vi "retraceSearchPath.vi"(8 "error in (no error)":errorcluster, 10 "GoalNode":refnum<data-value>, 11 "Graph in":refnum<class "Graph.lvclass">) -> (0 "error out":errorcluster, 2 "SearchPath":refnum<data-value>[](array[refnum]), 3 "Graph out":refnum<class "Graph.lvclass">)   [LabVIEW 2010, in "Graph.lvclass"]
doc: "At the end of a search, we retrace the path it took to reach the goal node."
uses:
  Graph.lvclass
  GraphNode/GraphNode.lvclass
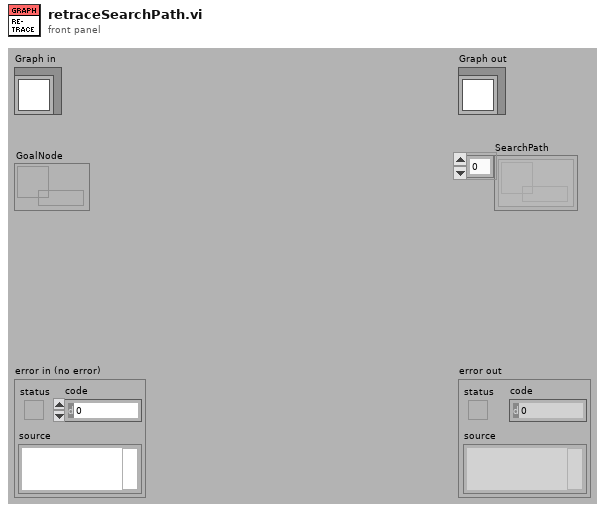
[diagram p1: front panel]
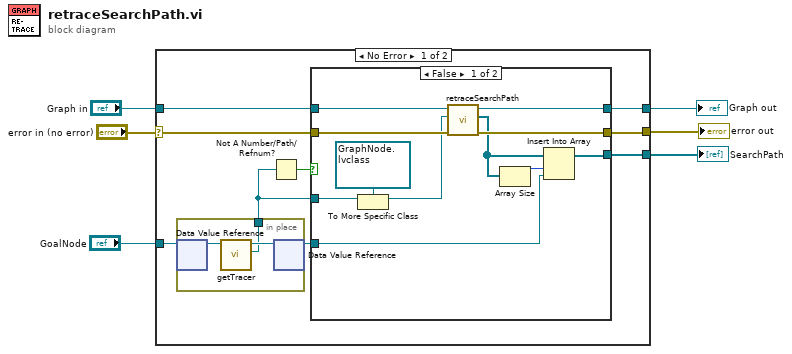
[diagram p0: block diagram]
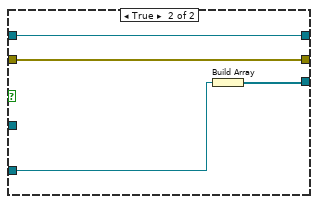
[diagram p2: hidden frame]
diagram:
  n1 = case shown="No Error" "error in (no error)" {
    selector: "error in (no error)" -> [w13 w35]
    tunnel: [w11 w35] -> w5
    tunnel: [w14 w34] -> w3
    tunnel: "Graph in" -> [w15 w34]
    tunnel: "GoalNode" -> [w12 _]
    tunnel: [w10 _] -> w1
    frame No Error {
      n2 = in-place {
        in-place-border: [w31] -> w7
        n3 = in-place-dvr #1(w12) -> (w33:refnum<class "GraphNode.lvclass">)  [unwired: 1 out]
        n4 = call "getTracer.vi"("GraphNode in"=w33) -> ("tracer"=w31:refnum<data-value>, "GraphNode out"=w32:refnum<class "GraphNode.lvclass">)  [unwired: 8 in, 1 out]
        n5 = in-place-dvr #1(w32) -> (w9:refnum<data-value>)  [unwired: 1 out]
      }
      n6 = Not A Number/Path/Refnum?(number/path/refnum=w7) -> (NaN/Path/Refnum?=w8:bool)
      n7 = case shown="False" w8 {
        tunnel: w15 -> [w26 w27]
        tunnel: [w25 w27] -> w14
        tunnel: w13 -> [w24 w28]
        tunnel: [w23 w28] -> w11
        tunnel: [w22 w29] -> w10
        tunnel: w9 -> [w19 w30]
        tunnel: w7 -> [w18 _]
        frame False {
          n8 = To More Specific Class(target class=refnum<data-value> refnum ("GoalNode"), reference=w18) -> (specific class reference=w20:refnum<data-value>)  [unwired: 1 in, 1 out]
          n9 = call "retraceSearchPath.vi"("error in (no error)"=w24, "GoalNode"=w20, "Graph in"=w26) -> ("error out"=w23:errorcluster, "SearchPath"=w17:refnum<data-value>[], "Graph out"=w25:refnum<class "Graph.lvclass">)  [unwired: 6 in]
          n10 = Array Size(array=w17) -> (size(s)=w16:i32)
          n11 = Insert Into Array(array=w17, index=w16, new element=w19) -> (w22:refnum<data-value>[])
        }
        frame True {
          n12 = Build Array(w30) -> (w29:refnum<data-value>[])
        }
      }
    }
    frame Error {
    }
  }
  "error out" <- w5
  "Graph out" <- w3
  "SearchPath" <- w1
